vi "getRevision.vi"() -> ()   [LabVIEW 2017]
uses:
  System.Drawing
  System.Windows.Forms
panel:
  out "revision":i32
  in  "URL":string="https://svn.cim.as/svn/CIM_TM/Projects/3173 SVS - SmartVisionSystem/LV2017/trunk"
  out "last change date":string
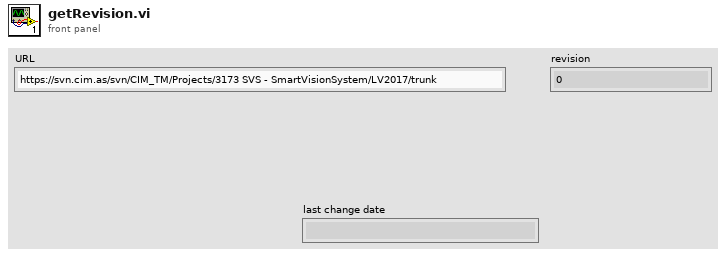
[diagram p1: front panel]
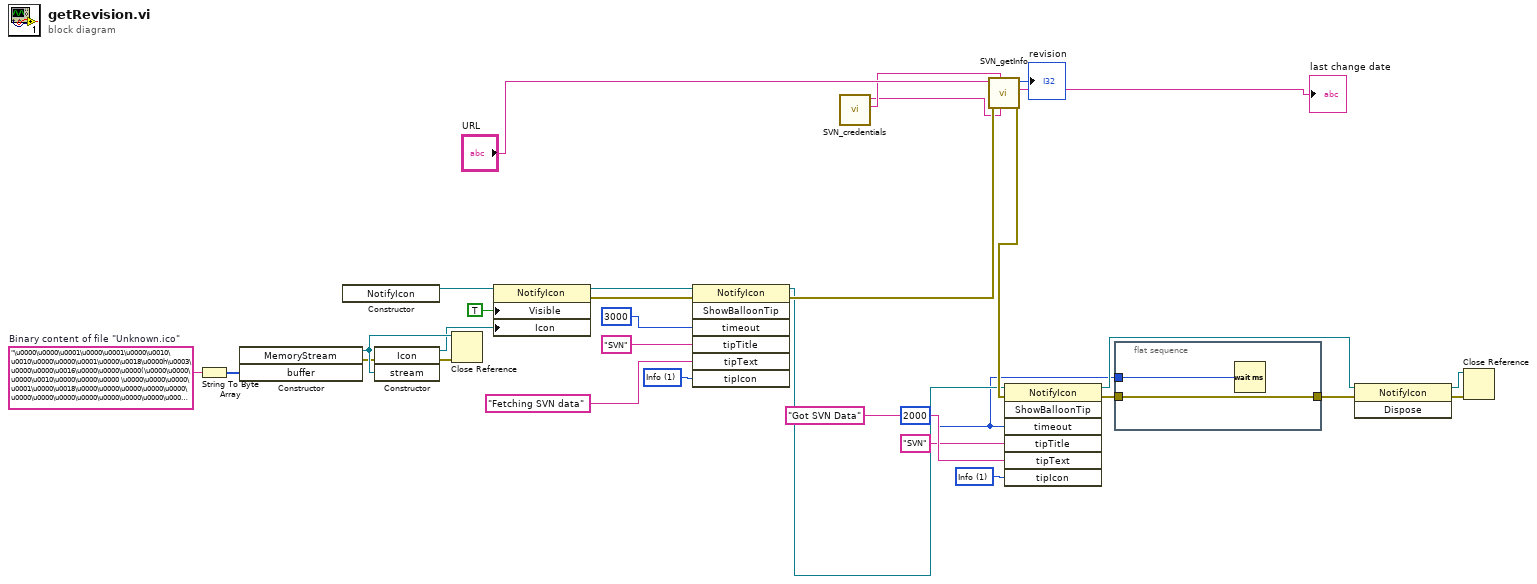
[diagram p0: block diagram]
diagram:
  w7 = "\u0000\u0000\u0001\u0000\u0001\u0000\u0010\u0010\u0000\u0000\u0001\u0000\u0018\u0000h\u0003\u0000\u0000\u0016\u0000\u0000\u0000(\u0000\u0000\u0000\u0010\u0000\u0000\u0000 \u0000\u0000\u0000\u0001\u0000\u0018\u0000\u0000\u0000\u0000\u0000\u0000\u0000\u0000\u0000\u0000\u0000\u0000\u0000\u0000\u0000\u0000\u0000\u0000\u0000\u0000\u0000\u0000\u0000\u0000\u0000ÿÿÿÿÿÿÿÿÿÿÿÿÿÿÿÿÿÿÿÿÿÿÿÿÿÿÿÿÿÿÿÿÿÿÿÿÿÿÿÿÿÿÿÿÿÿÿÿÿÿÿww}PPvFFvDDrBBp@@n==l;;k::k::k99j99k<<vvÿÿÿÿÿÿVV£xx]]__]]XX__WWOONN}JJxEEn;;j;;ÿÿÿÿÿÿ__­iikkgg½ùôôûîî¯}}YYWWQQxEEi88ÿÿÿÿÿÿcc´£pp£pphhË¾¾ùÿÿÿÿÿÖ³³^^\\\\WW}JJi88ÿÿÿÿÿÿhh»©uu©vv©vvcc·À¢llhhbb^^NNj99ÿÿÿÿÿÿkkÄ¯zz°}}¯{{¾Á¹¤oollggbbTTk::ÿÿÿÿÿÿppÉ¢¢¶¶´Ñ°°ÿÿÿÿÿÿÇ¡llkkhhWWn==ÿÿÿÿÿÿttÑ««¼¾¼¹øõõÿÿÿÿÿÿÜºº¢llii\\\\rAAÿÿÿÿÿÿ¡xxÖ±±ÃÄÅ²zz³zzõîîÿÿÿÿÿÿ·ll__sBBÿÿÿÿÿÿ¤||Ü¹¹ÉÇ«}}ÞÙÙÐ¸¸ðììúûûÿÿÿ» mm``vFFÿÿÿÿÿÿ§~~à¿¿Ì..."  # Binary content of file "Unknown.ico"
  w15 = 1 items=["None", "Info", "Warning", "Error"] ("tipIcon")
  w4 = 2000 ("timeout")
  w24 = 1 items=["None", "Info", "Warning", "Error"] ("tipIcon")
  n1 = String To Byte Array(string=w7) -> (unsigned byte array=w5:u8[])
  n2 = constructor class="MemoryStream"("buffer"=w5) -> (reference out=w18:refnum<k24>, error out=w17:errorcluster)  [unwired: 3 in, 2 out]
  n3 = constructor class="NotifyIcon"() -> (reference out=w23:refnum<k24>)  [unwired: 3 in, 2 out]
  n4 = constructor class="Icon"(error in=w17, "stream"=w18) -> (reference out=w6:refnum<k24>, error out=w19:errorcluster)  [unwired: 2 in, 2 out]
  n5 = Close Reference(reference=w18, error in (no error)=w19) -> ()  [unwired: 1 out]
  n6 = property class="NotifyIcon"(reference=w23, "Visible"=TRUE, "Icon"=w6) -> (reference out=w22:refnum<k24>, error out=w21:errorcluster)  [unwired: 1 in]
  n7 = invoke class="NotifyIcon" method="ShowBalloonTip"(reference=w22, error in=w21, "timeout"=3000, "tipTitle"="SVN", "tipText"="Fetching SVN data", "tipIcon"=w24) -> (reference out=w11:refnum<k24>, error out=w16:errorcluster)  [unwired: 1 in, 5 out]
  n8 = call "SVN_credentials.vi"() -> ("Username"=w2:string, "Password"=w1:string)  [unwired: 10 in]
  n9 = call "SVN_getInfo.vi"("password"=w1, "username"=w2, "error in (no error)"=w16, "URL"="URL") -> ("error out"=w12:errorcluster, "lastChangeDate"=→"last change date":string, "revision"=→"revision":i32)  [unwired: 5 in]
  n10 = invoke class="NotifyIcon" method="ShowBalloonTip"(reference=w11, error in=w12, "timeout"=w4, "tipTitle"="SVN", "tipText"="Got SVN Data", "tipIcon"=w15) -> (reference out=w8:refnum<k24>, error out=w9:errorcluster)  [unwired: 1 in, 5 out]
  n11 = flat-sequence {
    tunnel: [w33] -> w10
    tunnel: w9 -> [w33]
    tunnel: w4 -> [w32]
    frame #0 {
      n12 = Wait (ms)(milliseconds to wait=w32) -> ()  [unwired: 1 out]
    }
  }
  n13 = invoke class="NotifyIcon" method="Dispose"(reference=w8, error in=w10) -> (reference out=w28:refnum<k24>, error out=w29:errorcluster)  [unwired: 1 in, 1 out]
  n14 = Close Reference(reference=w28, error in (no error)=w29) -> ()  [unwired: 1 out]
